vi "ActionVIOnLoad.vi"(8 "error in (no error)":errorcluster, 11 "Device Item Ref in":T1 format="%.0x") -> (0 "error out":errorcluster, 3 "Device Item Ref out":T1 format="%.0x")   [LabVIEW 2020, in "Ballard MIL-STD-1553 System Explorer.lvlib"]
uses:
  Ballard MIL-STD-1553 System Explorer.lvlib
  <vilib>/NI VeriStand/Custom Device API/Custom Device Item Ref.ctl
  Includes/Ballard MIL-STD-1553 System Explorer.lvlibp/System Explorer/Implementation/Implementation.lvlib
  <vilib>/NI VeriStand/Custom Device API/Custom Device API.lvlib
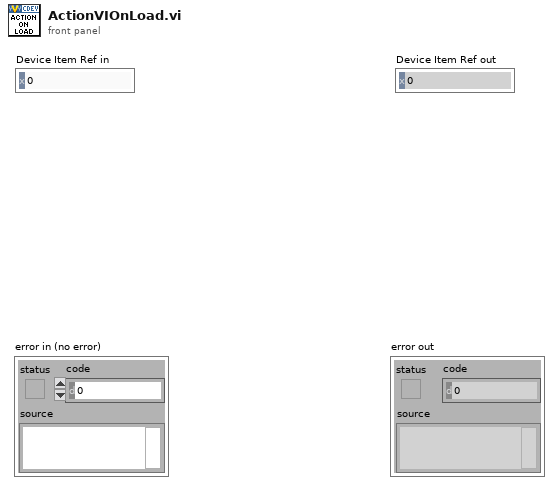
[diagram p1: front panel]
types:
  T1 = typedef "Custom Device API.lvlib/Custom Device Item Ref.ctl" = u64
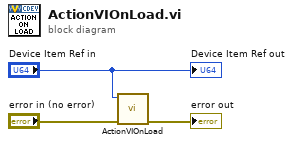
[diagram p0: block diagram]
diagram:
  n1 = call "ActionVIOnLoad.vi"("error in (no error)"="error in (no error)", "Device Item Ref in"="Device Item Ref in") -> ("error out"=→"error out":errorcluster)  [unwired: 8 in, 1 out]
  "Device Item Ref out" <- "Device Item Ref in"
